vi "Destroy to Session.vi"(8 "Error In":errorcluster, 10 "File Info":refnum<class "File Info.lvclass">, 11 "Session In":refnum<class "Session.lvclass">) -> (0 "Error Out":errorcluster, 3 "Session Out":refnum<class "Session.lvclass">)   [LabVIEW 2018, in "Toolkit.lvlib" / "File Info.lvclass"]
uses:
  File Info.lvclass
  Session/Session.lvclass
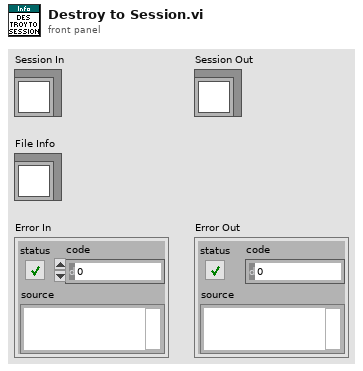
[diagram p1: front panel]
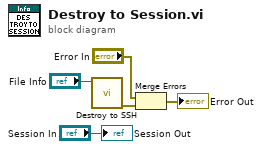
[diagram p0: block diagram]
diagram:
  n1 = call "Destroy to SSH.vi"("File Info"="File Info") -> ("Error Out"=w1:errorcluster)  [unwired: 9 in, 1 out]
  n2 = Merge Errors("Error In", w1) -> (→"Error Out":errorcluster)
  "Session Out" <- "Session In"
